vi "Deposit_Init.vi"(8 "error in (no error)":errorcluster, 11 "Deposit_Init in":refnum<class "Deposit_Init.lvclass">) -> (0 "error out":errorcluster, 3 "State out":refnum<class "State Actor.lvclass">)   [LabVIEW 2025, in "ATM_UI_Controller.lvlib" / "Deposit_Init.lvclass"]
uses:
  Deposit_Init.lvclass
  Deposit_Init.lvclass/Deposit_Init.ctl
  C:/Users/halstead_rideriver/Documents/Labview_Practice/ATM_Machine_Actor Framework/ATM_ACTORFW/ATM_UI_Controller/ATM_UI_Controller.lvclass
  C:/Program Files (x86)/National Instruments/LabVIEW 2025/vi.lib/ni/Actors/State Actor/State Actor/State Actor.lvclass
  C:/Program Files (x86)/National Instruments/LabVIEW 2025/vi.lib/ActorFramework/Actor/Actor.lvclass
  C:/Users/halstead_rideriver/Documents/Labview_Practice/ATM_Machine_Actor Framework/ATM_ACTORFW/ATM_UI_Controller/Deposit_Init/Deposit_Init.lvclass
  <vilib>/ni/Actors/State Actor/State Actor/State Actor.lvclass
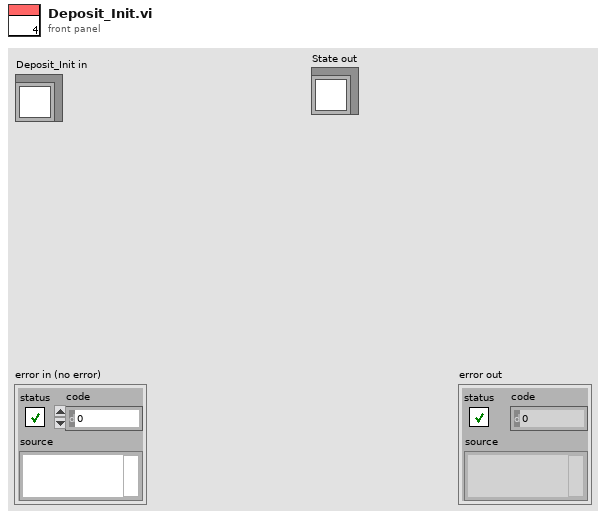
[diagram p1: front panel]
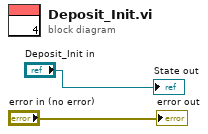
[diagram p0: block diagram]
diagram:
  "error out" <- "error in (no error)"
  "State out" <- "Deposit_Init in"
